vi "Point_Get_Datatype.vi"(8 "Error In":errorcluster, 10 "Tag":string, 11 "Map":T2) -> (0 "Error Out":errorcluster, 2 "Found?":bool, 3 "Map Out":T2, 4 "Datatype":T1)   [LabVIEW 2017, in "PointValueMap.lvlib"]
uses:
  <vilib>/addons/PointValueMap/PointValueMap.lvlib
  <vilib>/addons/PointValueMap/controls/PointMap.ctl
  <vilib>/addons/PointValueMap/controls/DataTypes.ctl
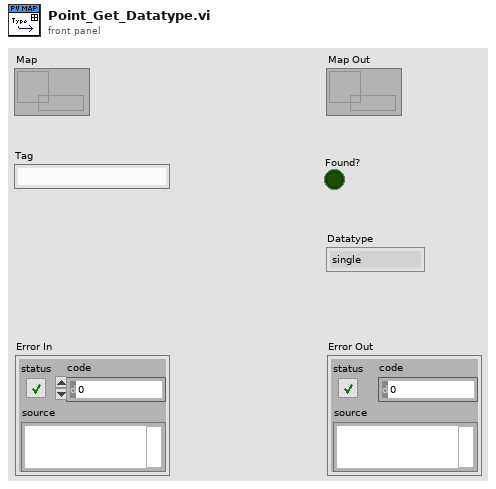
[diagram p1: front panel]
types:
  T1 = typedef "PointValueMap.lvlib/DataTypes.ctl" = enum16{"single", "double", "i32", "string", "variant"}
  T2 = typedef "PointValueMap.lvlib/PointMap.ctl" = refnum<data-value>
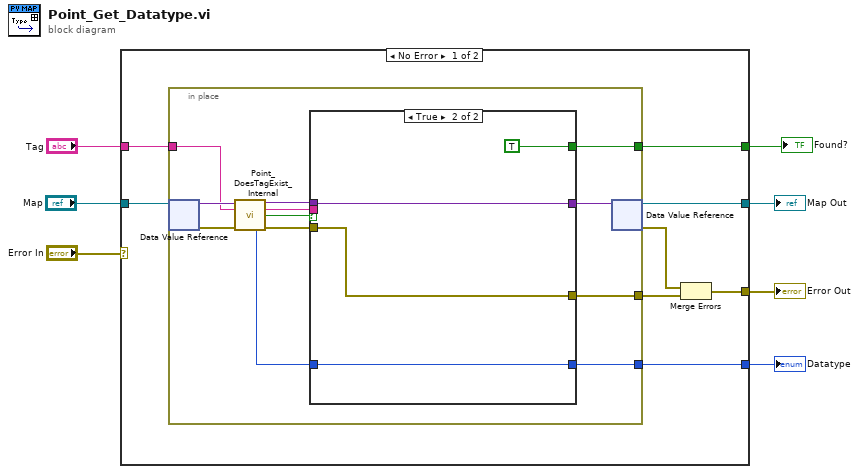
[diagram p0: block diagram]
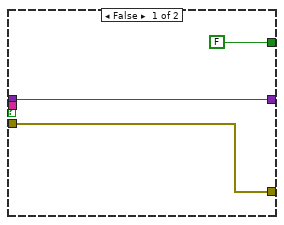
[diagram p2: hidden frame]
diagram:
  n1 = case shown="No Error" "Error In" {
    selector: "Error In" -> [_ w36]
    tunnel: "Map" -> [w15 w35]
    tunnel: "Tag" -> [w14 _]
    tunnel: [w11 w36] -> w6
    tunnel: [w10 _] -> w2
    tunnel: [w9 w35] -> w3
    tunnel: [w8 _] -> w1
    frame No Error {
      n2 = in-place {
        in-place-border: w14 -> [w19]
        in-place-border: [w26] -> w12
        in-place-border: [w25] -> w10
        in-place-border: [w16] -> w8
        n3 = in-place-dvr #1(w15) -> (w24:variant, w22:errorcluster)
        n4 = call <vilib>:"Point_DoesTagExist_Internal.vi"("Map"=w24, "Tag"=w19, "Error In"=w22) -> ("Map Out"=w23:variant, "Tag Out"=w18:string, "Tag Exists"=w20:bool, "Datatype"=w17:T1, "Error Out"=w21:errorcluster)  [unwired: 7 in, 1 out]
        n5 = case shown="True" w20 {
          tunnel: [w30 w33] -> w27
          tunnel: [w28 w32] -> w26
          tunnel: [_ w34] -> w25
          tunnel: w23 -> [w30 w33]
          tunnel: w21 -> [w28 w32]
          tunnel: w18 -> [_ _]
          tunnel: w17 -> [_ w34]
          tunnel: [FALSE TRUE] -> w16
          frame False {
          }
          frame True {
          }
        }
        n6 = in-place-dvr #1(w27) -> (w9:T2, w13:errorcluster)
      }
      n7 = Merge Errors(w13, w12) -> (w11:errorcluster)
    }
    frame Error {
    }
  }
  "Error Out" <- w6
  "Map Out" <- w3
  "Datatype" <- w2
  "Found?" <- w1
